vi "Read VI Reference.vi"(8 "error in (no error)":errorcluster, 11 "UI Reference Wrapper in":refnum<class "UI Reference Wrapper.lvclass">) -> (0 "error out":errorcluster, 2 "VI Reference Wrappers":cluster{"VI Refnum":refnum<vi>, "Name":string}[](array[cluster]), 3 "UI Reference Wrapper out":refnum<class "UI Reference Wrapper.lvclass">)   [LabVIEW 2019, in "UI Reference Wrapper.lvclass"]
uses:
  UI Reference Wrapper.lvclass
  UI Reference Wrapper.lvclass/UI Reference Wrapper.ctl
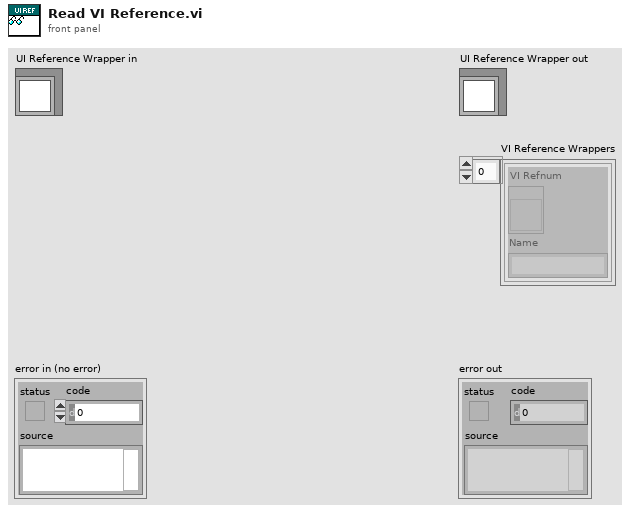
[diagram p1: front panel]
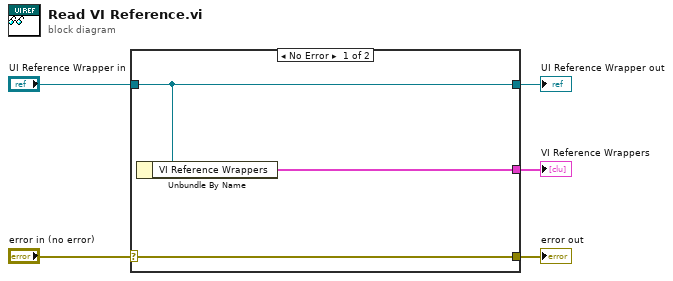
[diagram p0: block diagram]
diagram:
  n1 = case shown="No Error" "error in (no error)" {
    selector: "error in (no error)" -> [w8 w9]
    tunnel: [w8 w9] -> w4
    tunnel: [w7 w10] -> w2
    tunnel: "UI Reference Wrapper in" -> [w7 w10]
    tunnel: [w6 _] -> w1
    frame No Error {
      n2 = Unbundle By Name(w7) -> ("VI Reference Wrappers"=w6:cluster{"VI Refnum":refnum<vi>, "Name":string}[])
    }
    frame Error {
    }
  }
  "error out" <- w4
  "UI Reference Wrapper out" <- w2
  "VI Reference Wrappers" <- w1
